vi "Close Instrument.vi"(7 "Go Local (\"@LOC\")":bool, 8 "error in (no error)":errorcluster, 11 "VNA-ENA in":refnum<class "VNA-ENA.lvclass">) -> (0 "error out":errorcluster, 3 "VNA-ENA out":refnum<class "VNA-ENA.lvclass">)   [LabVIEW 2020, in "VNA-ENA.lvclass"]
uses:
  VNA-ENA.lvclass
  C:/Sandbox/RF Bench/Source Code/WiSpry Test Framework/Instruments/Instrument.lvclass
  Instrument.lvclass/Instrument.ctl
  Vector Network Analyzer.lvclass
  <instrlib>/Agilent ENA Series/Agilent ENA Series.lvlib
  Instrument.lvclass
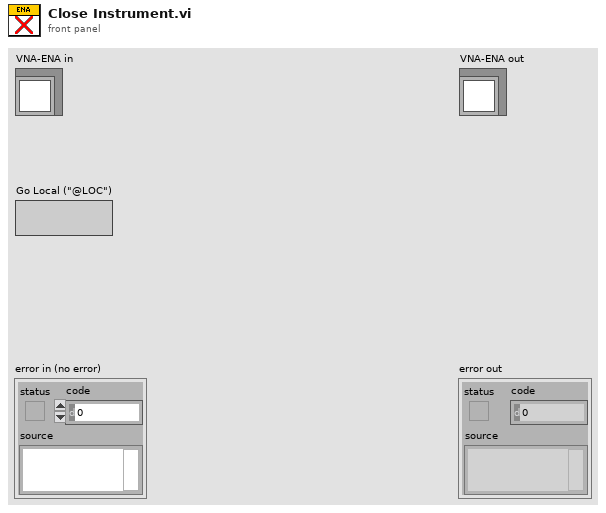
[diagram p1: front panel]
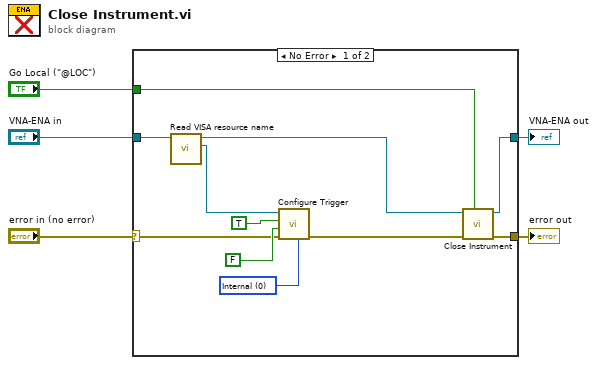
[diagram p0: block diagram]
diagram:
  n1 = case shown="No Error" "error in (no error)" {
    selector: "error in (no error)" -> [w10 w18]
    tunnel: [w16 w18] -> w5
    tunnel: [w15 w17] -> w4
    tunnel: "Go Local (\"@LOC\")" -> [w14 _]
    tunnel: "VNA-ENA in" -> [w9 w17]
    frame No Error {
      w11 = u16 0 items=["Internal", "External", "Manual", "BUS"] ("Trigger Source (0: Internal)")
      n2 = call "Read VISA resource name.vi"("Instrument in"=w9) -> ("VISA resource name"=w7:refnum<visa-resource-name>, "Instrument out"=w8:refnum<class "VNA-ENA.lvclass">)  [unwired: 9 in]
      n3 = call <instrlib>:"Configure Trigger.vi"("Trigger Source (0: Internal)"=w11, "error in (no error)"=w10, "Point Trigger (F: Disable)"=FALSE, "Continuous Sweep (T: Enable)"=TRUE, "VISA resource name"=w7) -> ("error out"=w6:errorcluster)  [unwired: 5 in, 1 out]
      n4 = call-parent "Close Instrument.vi"("Go Local (\"@LOC\")"=w14, "error in (no error)"=w6, "Instrument in"=w8) -> ("error out"=w16:errorcluster, "Instrument out"=w15:refnum<class "VNA-ENA.lvclass">)  [unwired: 7 in]
    }
    frame Error {
    }
  }
  "error out" <- w5
  "VNA-ENA out" <- w4
